vi "Stand Alone Display Main.vi"(8 "error in (no error)":errorcluster, 11 "Stand Alone Display Actor in":refnum<class "Stand Alone Display Actor.lvclass">) -> (0 "error out":errorcluster, 3 "Stand Alone Display Actor out":refnum<class "Stand Alone Display Actor.lvclass">)   [LabVIEW 2024, in "Stand Alone Display Actor.lvclass"]
uses:
  Stand Alone Display Actor.lvclass
  Ancestor Class/Actor/System Actor/Public Data/Read Actor Name.vi
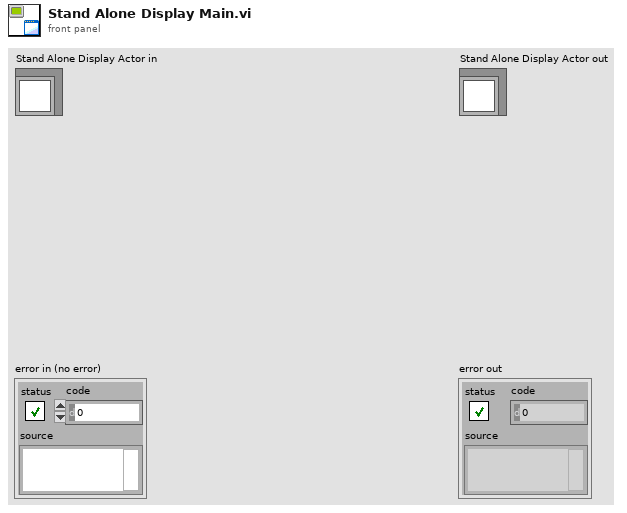
[diagram p1: front panel]
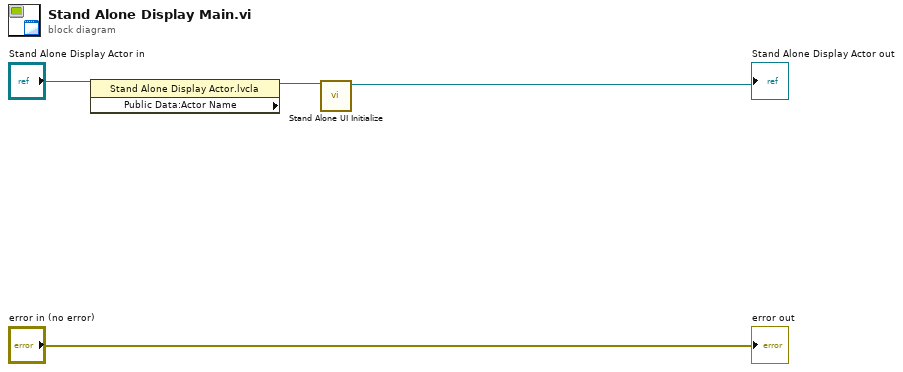
[diagram p0: block diagram]
diagram:
  n1 = property class="Stand Alone Display Actor.lvcla" props=["Public Data:Actor Name"](reference="Stand Alone Display Actor in") -> (reference out=w2:refnum<class "Stand Alone Display Actor.lvclass">)  [unwired: 1 in, 2 out]
  n2 = call-dynamic "Stand Alone UI Initialize.vi"("Stand Alone Display Actor in"=w2) -> ("Stand Alone Display Actor out"=→"Stand Alone Display Actor out":refnum<class "Stand Alone Display Actor.lvclass">)  [unwired: 9 in, 1 out]
  "error out" <- "error in (no error)"
